vi "ISEG_HVSystemGUI.appendTimeStampString.vi"(2 "error in":errorcluster, 3 "String":string) -> (0 "error out":errorcluster, 1 "String with TS":string)   [LabVIEW 2014, in "ISEG_HVSystemGUI.lvlib"]
doc: "This VI appends a timestamp string to the input string."
uses:
  ISEG_HVSystemGUI.lvlib
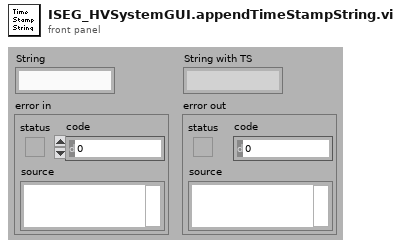
[diagram p1: front panel]
types:
  T1 = typedef "LVDateTimeRec.ctl" = cluster{"fractional second":dbl, "second":i32, "minute":i32, "hour":i32, "day of month":i32, "month":i32, "year":i32, "day of week":i32, "day of year":i32, "DST":i32}
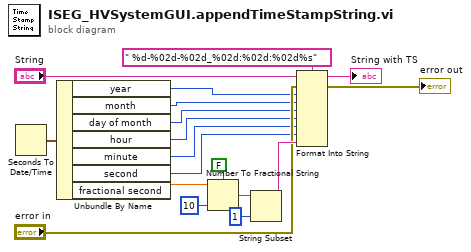
[diagram p0: block diagram]
diagram:
  n1 = Seconds To Date/Time() -> (date time rec=w1:T1)  [unwired: 2 out]
  n2 = Unbundle By Name(w1) -> ("year"=w2:i32, "month"=w3:i32, "day of month"=w4:i32, "hour"=w5:i32, "minute"=w6:i32, "second"=w7:i32, "fractional second"=w10:dbl)
  n3 = Number To Fractional String(use system decimal point (T)=FALSE, number=w10, precision (6)=i16 10) -> (F-format string=w17:string)  [unwired: 1 out]
  n4 = String Subset(string=w17, offset (0)=1) -> (substring=w18:string)  [unwired: 1 out]
  n5 = Format Into String(format string=" %d-%02d-%02d_%02d:%02d:%02d%s", initial string="String", error in="error in", w2, w3, w4, w5, w6, w7, w18) -> (resulting string=→"String with TS":string, error out=→"error out":errorcluster)
